vi "Replace Root.vi"(11 "Map in":map{string, string}(c390)) -> (3 "Map out":map{string, string}(c390))   [LabVIEW 2021]
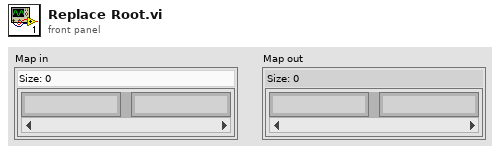
[diagram p1: front panel]
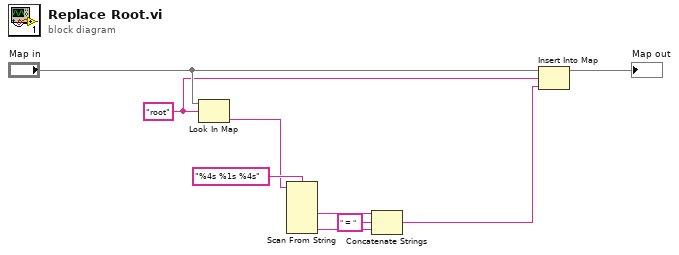
[diagram p0: block diagram]
diagram:
  w1 = "root" ("key")
  n1 = Look In Map(map="Map in", key=w1) -> (value=w6:string)  [unwired: 1 in, 1 out]
  n2 = Scan From String(format string="%4s %1s %4s", input string=w6) -> (output 1=w5:string, output 3=w4:string)  [unwired: 6 in, 3 out]
  n3 = Concatenate Strings(w5, " = " ("string"), w4) -> (w2:string)
  n4 = Insert Into Map(map in="Map in", key=w1, value=w2) -> (map out=→"Map out":map{string, string})  [unwired: 2 out]
